vi "Read Current Cell.vi"(8 "error in":errorcluster, 11 "PAS Data in":refnum<class "PAS Data.lvclass">) -> (0 "error out":errorcluster, 2 "Current Cell":i32, 3 "PAS Data out":refnum<class "PAS Data.lvclass">)   [LabVIEW 2015, in "PAS Data.lvclass"]
uses:
  PAS Data.lvclass
  PAS Data.lvclass/PAS Data.ctl
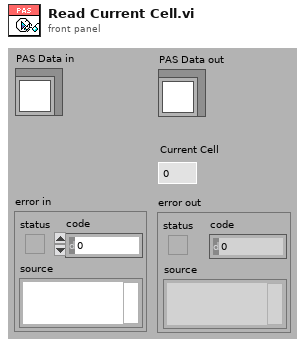
[diagram p1: front panel]
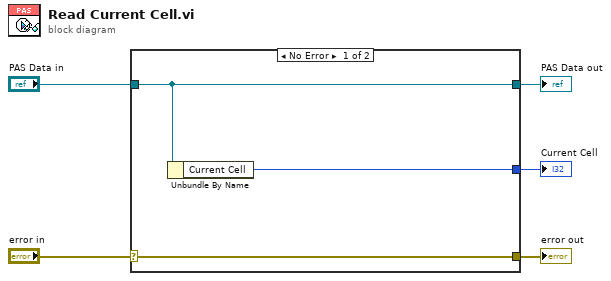
[diagram p0: block diagram]
diagram:
  n1 = case shown="No Error" "error in" {
    selector: "error in" -> [w8 w9]
    tunnel: [w8 w9] -> w4
    tunnel: [w7 w10] -> w2
    tunnel: "PAS Data in" -> [w7 w10]
    tunnel: [w6 _] -> w1
    frame No Error {
      n2 = Unbundle By Name(w7) -> ("Current Cell"=w6:i32)
    }
    frame Error {
    }
  }
  "error out" <- w4
  "PAS Data out" <- w2
  "Current Cell" <- w1
